vi "ComputeCOM.vi"(0 "tracker":u64, 1 "median":sgl=-1.0) -> (2 "tracker":u64, 3 "median":sgl, 4 "position":cluster{"X":sgl, "Y":sgl})   [LabVIEW 2011]
uses:
  TrackerDLL.vi
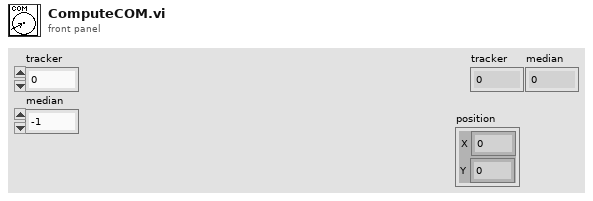
[diagram p1: front panel]
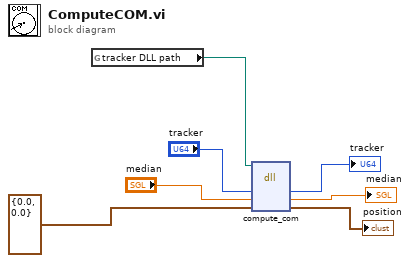
[diagram p0: block diagram]
diagram:
  n1 = global read "TrackerDLL.vi" "tracker DLL path"() -> (w3:path)
  n2 = dll-call lib="D:/jcnossen1/cudaqi-tracker/cudatrack-labview/cputrack.dll" fn="compute_com"(path in=w3, "tracker"="tracker", "median"="median", "position"=cluster{sgl, sgl} {0.0, 0.0}) -> ("tracker"=→"tracker":u64, "median"=→"median":sgl, "position"=→"position":cluster{sgl, sgl})  [unwired: 3 in, 2 out]
